vi "Example.vi"() -> ()   [LabVIEW 2016]
panel:
  in  "stop":bool
  in  "Boolean":bool
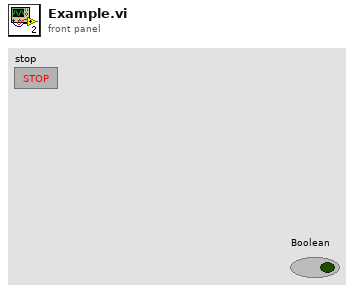
[diagram p1: front panel]
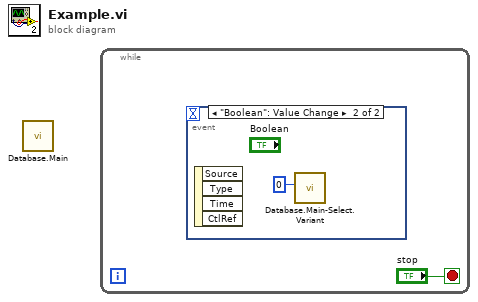
[diagram p0: block diagram]
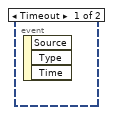
[diagram p2: hidden frame]
diagram:
  n1 = call "Database.Main.vi"() -> ()  [unwired: 1 in]
  n2 = while {
    stop <- "stop" stop-if-true
    n3 = event shown="[1] \"Boolean\": Value Change" {
      selector: _ -> [_ _]
      dyn-events: _ -> [_ _]
      timeout: _ -> [_ _]
      event Timeout {
        n4 = event-data() -> ()  [unwired: 1 in, 3 out]
      }
      event "Boolean": Value Change {
        n5 = event-data() -> ()  [unwired: 1 in, 4 out]
        n6 = call "Database.Main-Select.Variant.vi"("SelectVariant Format"=u64 0 ("Variant Ref")) -> ()  [unwired: 10 in, 1 out]
      }
    }
  }
